vi "solar_app Splash Screen.vi"(4 "AppSetup":string="N/A" caption="Application Setup:", 6 "PartNumber":string="N/A" caption="Part Number:", 8 "SOLARVersion":string="N/A" caption="Version:", 9 "ExeVersion":string="N/A" caption="Application Version:", 10 "SplashPath":string, 11 "SplashWait":i32) -> ()   [LabVIEW 2018]
doc: "This is the splash screen displayed."
panel:
  in  "Destroy":bool
  in  "Exit":bool
  in  "Info":string
  out "Click":string="Click in window to continue"
  out "Image":picture
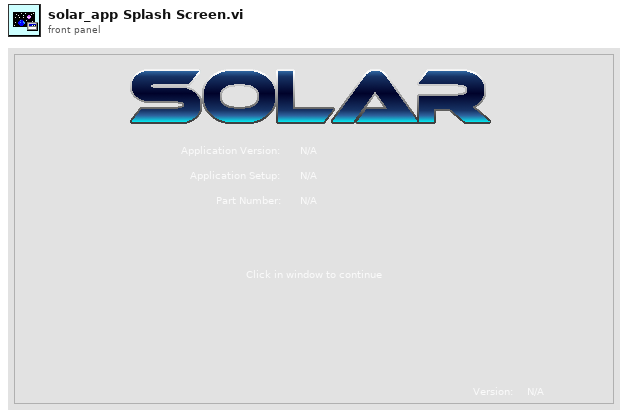
[diagram p1: front panel]
types:
  T1 = typedef "imagedata.ctl" = cluster{"image type":i32, "image depth":i32, "image":u8[], "mask":u8[], "colors":u32[], "Rectangle":cluster{"left":i16, "top":i16, "right":i16, "bottom":i16}}
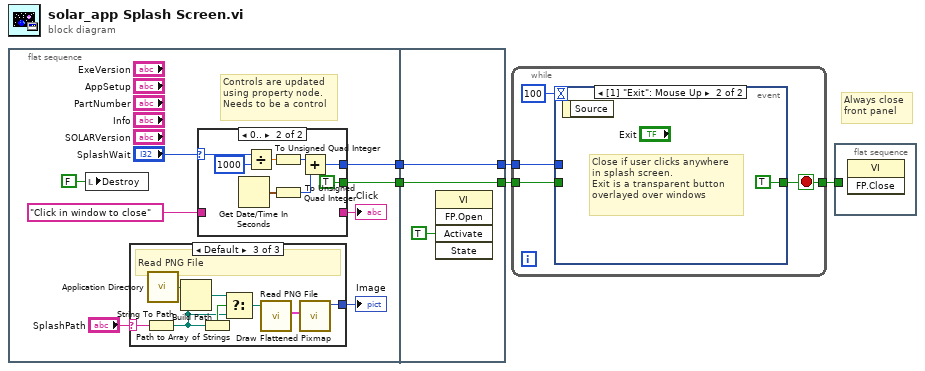
[diagram p0: block diagram]
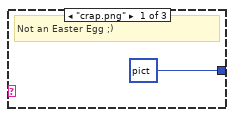
[diagram p2: hidden frame]
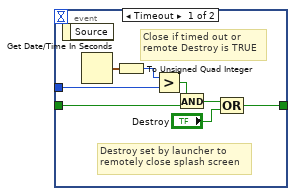
[diagram p5: hidden frame]
diagram:
  # "Always close\nfront panel"
  n1 = flat-sequence {
    tunnel: [w12] -> w2
    tunnel: [w10] -> w1
    tunnel: [w33] -> w3
    tunnel: [w34] -> w4
    tunnel: w2 -> [w34]
    tunnel: w1 -> [w33]
    frame #0 {
      # "Controls are updated\nusing property node.\nNeeds to be a control"
      n2 = local write "Destroy"(FALSE ("Destroy")) -> ()
      n3 = case shown="Default" "SplashPath" {
        selector: "SplashPath" -> [_ _ w16]
        tunnel: [picture bytes[656630] ("new picture") _ w21] -> w9
        frame "crap.png" {
          # "Not an Easter Egg ;)"
        }
        frame "" {
        }
        frame Default {
          # "Read PNG File"
          n4 = String To Path(string=w16) -> (path=w17:path)
          n5 = call <vilib>:"Application Directory.vi"() -> ("Application Directory"=w20:path)
          n6 = Build Path(base path=w20, name or relative path=w17) -> (appended path=w18:path)
          n7 = Path to Array of Strings(0:w17) -> (1:w19:bool)  [unwired: 1 out]
          n8 = Select(t=w18, s=w19, f=w17) -> (s? t:f=w15:path)
          n9 = call <vilib>:"Read PNG File.vi"("path to PNG file"=w15) -> ("image data"=w22:T1)  [unwired: 8 in, 2 out]
          n10 = call <vilib>:"Draw Flattened Pixmap.vi"("image data"=w22) -> ("new picture"=w21:picture)  [unwired: 8 in]
        }
      }
      "Image" <- w9
      n11 = case shown="0.." "SplashWait" {
        selector: "SplashWait" -> [_ w27]
        tunnel: [_ w29] -> w12
        tunnel: [w23 _] -> w11
        tunnel: "Click in window to close" ("Click") -> [w23 _]
        tunnel: [_ TRUE] -> w10
        frame ..-1 {
        }
        frame 0.. {
          n12 = Get Date/Time In Seconds() -> (seconds since 1Jan1904=w28:timestamp)
          n13 = Divide(x=w27, y=1000) -> (x/y=w25:dbl)
          n14 = To Unsigned Quad Integer(1:w25) -> (0:w30:u64)
          n15 = To Unsigned Quad Integer(1:w28) -> (0:w31:u64)
          n16 = Add(x=w30, y=w31) -> (x+y=w29:u64)
        }
      }
      "Click" <- w11
    }
    frame #1 {
      n17 = invoke class="VI" method="FP.Open"("Activate"=TRUE ("Activate?")) -> ()  [unwired: 4 in, 5 out]
    }
  }
  n18 = while {
    tunnel: [w36] -> w5
    tunnel: w4 -> [w38]
    tunnel: w3 -> [w37]
    stop <- w36 stop-if-true
    n19 = event shown="[1] \"Exit\": Mouse Up" {
      selector: _ -> [_ _]
      dyn-events: _ -> [_ _]
      timeout: 100 -> [_ _]
      tunnel: w38 -> [w46 _]
      tunnel: w37 -> [w40 _]
      tunnel: [w39 TRUE] -> w36
      event Timeout {
        # "Close if timed out or\nremote Destroy is TRUE"
        # "Destroy set by launcher to\nremotely close splash screen"
        n20 = event-data() -> ()  [unwired: 1 in, 1 out]
        n21 = Get Date/Time In Seconds() -> (seconds since 1Jan1904=w45:timestamp)
        n22 = To Unsigned Quad Integer(1:w45) -> (0:w44:u64)
        n23 = Greater?(x=w44, y=w46) -> (0:w42:bool)
        n24 = And(x=w42, y=w40) -> (x .and. y?=w41:bool)
        n25 = Compound Arithmetic op=OR(w41, "Destroy") -> (w39:bool)
      }
      event "Exit": Mouse Up {
        # "Close if user clicks anywhere\nin splash screen.\nExit is a transparent button\noverlayed over windows"
        n26 = event-data() -> ()  [unwired: 1 in, 1 out]
      }
    }
  }
  n27 = flat-sequence {
    tunnel: w5 -> [_]
    frame #0 {
      n28 = invoke class="VI" method="FP.Close"() -> ()  [unwired: 3 in, 3 out]
    }
  }
